vi "Example - G560.vi"() -> ()   [LabVIEW 2022 SP3]
uses:
  API/Public/TypeDefs/Speaker Lighting Zones.ctl
  API/Logitech Devices.lvlib
panel:
  in  "Front Right Color":u32(colorbox)
  in  "Rear Right Color":u32(colorbox)
  in  "Front Left Color":u32(colorbox)
  in  "Rear Left Color":u32(colorbox)
  # "Logitech G560"
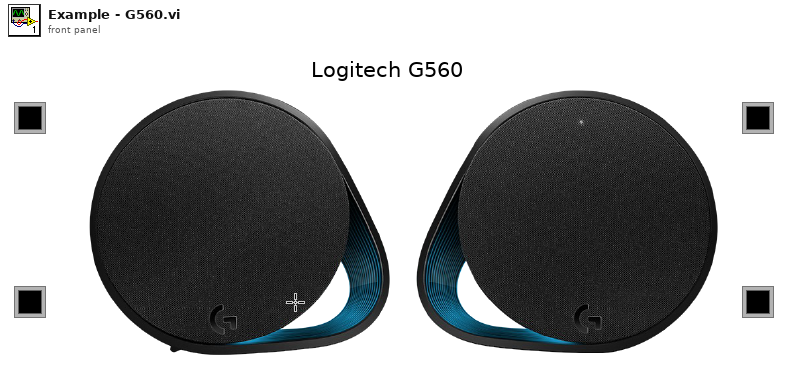
[diagram p1: front panel]
types:
  T1 = typedef "Logitech Devices.lvlib/Speaker Lighting Zones.ctl" = enum8{"Front left", "Front right", "Rear left", "Rear right"}
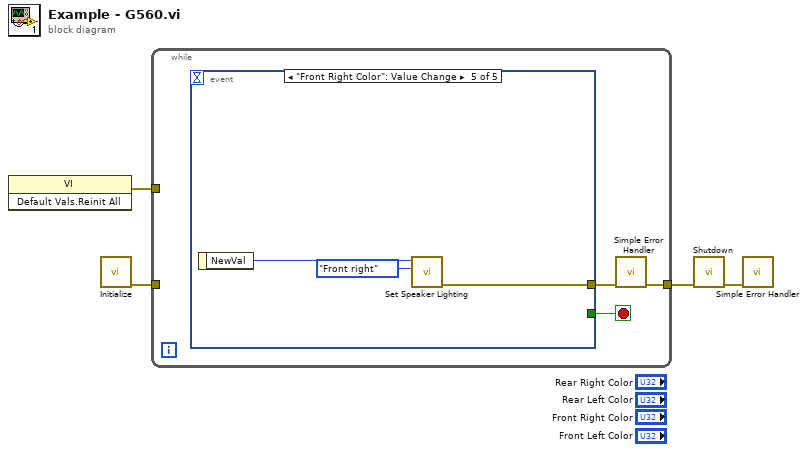
[diagram p0: block diagram]
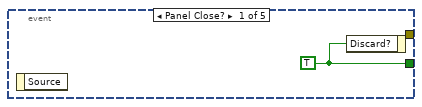
[diagram p2: hidden frame]
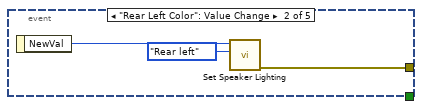
[diagram p3: hidden frame]
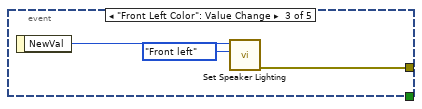
[diagram p4: hidden frame]
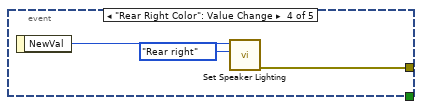
[diagram p5: hidden frame]
diagram:
  n1 = invoke class="VI" method="Default Vals.Reinit All"() -> (error out=w1:errorcluster)  [unwired: 3 in, 2 out]
  n2 = call "Initialize.vi"() -> ("error out"=w4:errorcluster)  [unwired: 11 in]
  n3 = while {
    tunnel: [w5] -> w3
    tunnel: w4 -> [_]
    tunnel: w1 -> [_]
    stop <- w7 stop-if-true
    n4 = event shown="[4] \"Front Right Color\": Value Change" {
      selector: _ -> [_ _ _ _ _]
      dyn-events: _ -> [_ _ _ _ _]
      timeout: _ -> [_ _ _ _ _]
      tunnel: [w8 _ _ _ _] -> w7
      tunnel: [_ w11 w14 w17 w20] -> w6
      event Panel Close? {
        w8 = TRUE
        n5 = event-data() -> ()  [unwired: 1 in, 1 out]
        n6 = event-data("Discard?"=w8) -> ()  [unwired: 1 in, 1 out]
      }
      event "Rear Left Color": Value Change {
        n7 = event-data() -> ("NewVal"=w10:u32)  [unwired: 1 in]
        n8 = call "Set Speaker Lighting.vi"("Lighting Zone"=Speaker_Lighting_Zones."Rear left", "LED Color"=w10) -> ("error out"=w11:errorcluster)  [unwired: 9 in]
      }
      event "Front Left Color": Value Change {
        n9 = event-data() -> ("NewVal"=w13:u32)  [unwired: 1 in]
        n10 = call "Set Speaker Lighting.vi"("Lighting Zone"=Speaker_Lighting_Zones."Front left", "LED Color"=w13) -> ("error out"=w14:errorcluster)  [unwired: 9 in]
      }
      event "Rear Right Color": Value Change {
        n11 = event-data() -> ("NewVal"=w16:u32)  [unwired: 1 in]
        n12 = call "Set Speaker Lighting.vi"("Lighting Zone"=Speaker_Lighting_Zones."Rear right", "LED Color"=w16) -> ("error out"=w17:errorcluster)  [unwired: 9 in]
      }
      event "Front Right Color": Value Change {
        n13 = event-data() -> ("NewVal"=w19:u32)  [unwired: 1 in]
        n14 = call "Set Speaker Lighting.vi"("Lighting Zone"=Speaker_Lighting_Zones."Front right", "LED Color"=w19) -> ("error out"=w20:errorcluster)  [unwired: 9 in]
      }
    }
    n15 = call <vilib>:"Simple Error Handler.vi"("error in (no error)"=w6) -> ("error out"=w5:errorcluster)  [unwired: 4 in, 4 out]
  }
  n16 = call "Shutdown.vi"("error in (no error)"=w3) -> ("error out"=w2:errorcluster)  [unwired: 10 in]
  n17 = call <vilib>:"Simple Error Handler.vi"("error in (no error)"=w2) -> ()  [unwired: 4 in, 5 out]
